vi "3_5_4.vi"() -> ()   [LabVIEW 2012]
panel:
  out "Array 3":i32[][](array[numeric])
  in  "Numeric":i32
  in  "Array 2":u8[][](array[numeric])
  in  "stop":bool
  in  "OK Button":bool
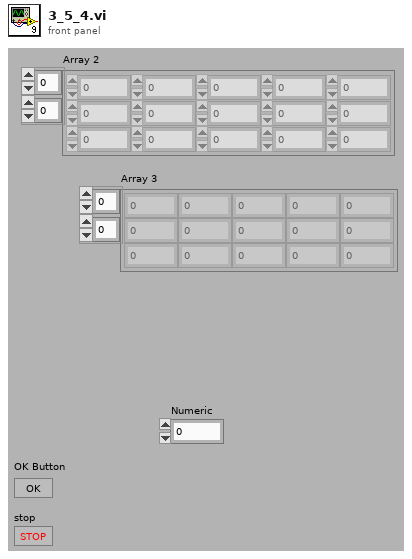
[diagram p1: front panel]
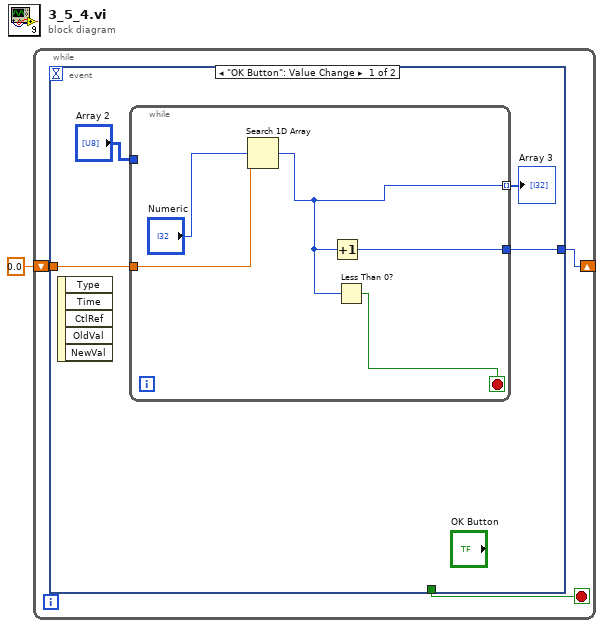
[diagram p0: block diagram]
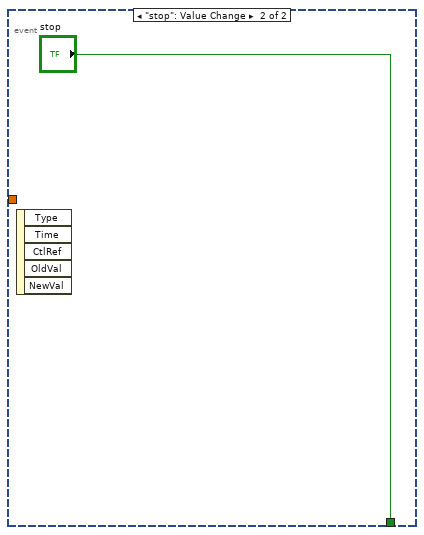
[diagram p2: hidden frame]
diagram:
  n1 = while {
    shift-right: [w4] -> _
    shift-left: 0.0 -> [w2]
    stop <- w3 stop-if-true
    n2 = event shown="[0] \"OK Button\": Value Change" {
      selector: _ -> [_ _]
      dyn-events: _ -> [_ _]
      timeout: _ -> [_ _]
      tunnel: [_ "stop"] -> w3
      tunnel: [w8 _] -> w4
      tunnel: w2 -> [w7 _]
      event "OK Button": Value Change {
        n3 = event-data() -> ()  [unwired: 1 in, 5 out]
        n4 = while {
          tunnel: [w13] -> w8
          tunnel: w7 -> [w11]
          tunnel: "Array 2" -> [_]
          tunnel: [w9] -> w5 mode=indexing
          stop <- w12 stop-if-true
          n5 = Search 1D Array(element="Numeric", start index (0)=w11) -> (index of element=w9:i32)  [unwired: 1 in]
          n6 = Increment(x=w9) -> (x+1=w13:i32)
          n7 = Less Than 0?(x=w9) -> (x < 0?=w12:bool)
        }
        "Array 3" <- w5
      }
      event "stop": Value Change {
        n8 = event-data() -> ()  [unwired: 1 in, 5 out]
      }
    }
  }
